vi "S2DS_Add path Extensipon.vi"(8 "Extension":string=".dat", 11 "path":path) -> (3 "Path":path)   [LabVIEW 2025]
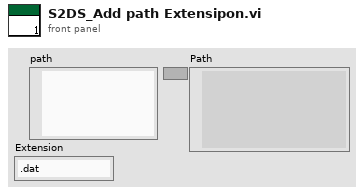
[diagram p1: front panel]
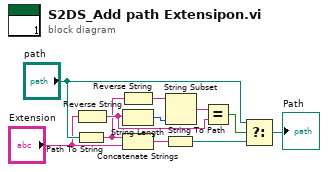
[diagram p0: block diagram]
diagram:
  n1 = Path To String(path="path") -> (string=w5:string)
  n2 = Reverse String(1:"Extension") -> (0:w8:string)
  n3 = Reverse String(1:w5) -> (0:w11:string)
  n4 = String Length(string=w8) -> (length=w10:i32)
  n5 = Concatenate Strings(w5, "Extension") -> (w3:string)
  n6 = String To Path(string=w3) -> (path=w2:path)
  n7 = String Subset(string=w11, length (rest)=w10) -> (substring=w9:string)  [unwired: 1 in]
  n8 = Equal?(x=w9, y=w8) -> (x = y?=w7:bool)
  n9 = Select(t="path", s=w7, f=w2) -> (s? t:f=→"Path":path)
